vi "Get Instrument Info Array from Connection Map for Each Site.vi"(10 "Pin Names for Scope":string[](array[string]), 11 "connection map":map{string, T1[]}(c390)) -> (3 "instrument info array for each site":T1[][](array[typedef]))   [LabVIEW 2021, in "PMIC Common.lvlib"]
uses:
  PMIC Common.lvlib
  Instrument Info.ctl
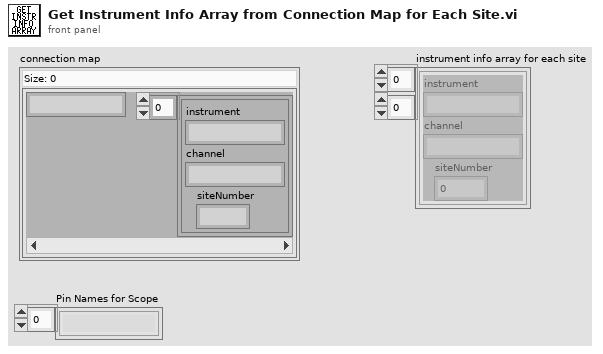
[diagram p1: front panel]
types:
  T1 = typedef "PMIC Common.lvlib/Instrument Info.ctl" = cluster{"instrument":string, "channel":string, "siteNumber":i32}
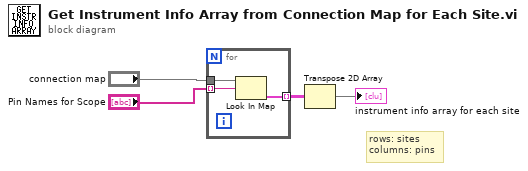
[diagram p0: block diagram]
diagram:
  # "rows: sites\ncolumns: pins"
  n1 = for {
    tunnel: "connection map" -> [w7]
    tunnel: "Pin Names for Scope" -> [w6] mode=indexing
    tunnel: [w5] -> w2 mode=indexing
    n2 = Look In Map(map=w7, key=w6) -> (value=w5:T1[])  [unwired: 1 in, 1 out]
  }
  n3 = Transpose 2D Array(2D array=w2) -> (transposed array=→"instrument info array for each site":T1[][])
